vi "Split_Ch_name.vi"(0 "Ch name":string) -> (1 "Top level":string, 2 "Middle":string, 3 "Low level":string)   [LabVIEW 2020]
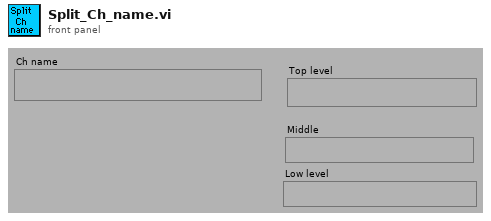
[diagram p1: front panel]
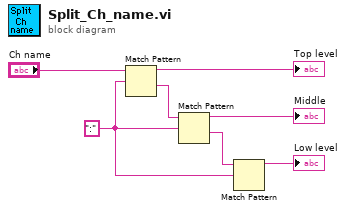
[diagram p0: block diagram]
diagram:
  w1 = ":" ("regular expression")
  n1 = Match Pattern(string="Ch name", regular expression=w1) -> (before substring=→"Top level":string, after substring=w6:string)  [unwired: 3 out]
  n2 = Match Pattern(string=w6, regular expression=w1) -> (before substring=→"Middle":string, after substring=w3:string)  [unwired: 3 out]
  n3 = Match Pattern(string=w3, regular expression=w1) -> (before substring=→"Low level":string)  [unwired: 4 out]
